vi "量程参数读取.vi"(8 "error in (no error)":errorcluster, 9 "量程下拉列表":enum16{"低量程", "高量程"}(ring), 10 "测量模式":enum16{"跨度核查", "水样测量", "零点核查", "标样核查", "加标回收"}(ring), 11 "参数下拉列表":u16(ring) items=["总磷"=1, "总氮"=2]) -> (0 "error out":errorcluster, 3 "量程切换阈值":cluster{"阈值":dbl, "标液浓度":dbl})   [LabVIEW 2016, in "斯坦道氨氮V2.lvlib"]
uses:
  <vilib>/Utility/error.llb/Error Cluster From Error Code.vi
  <vilib>/ErrorRing/Error Ring.xnode
  <vilib>/Plasmionique/MB Master/MB Master.lvlib
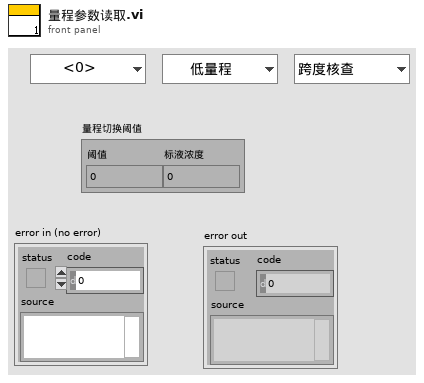
[diagram p1: front panel]
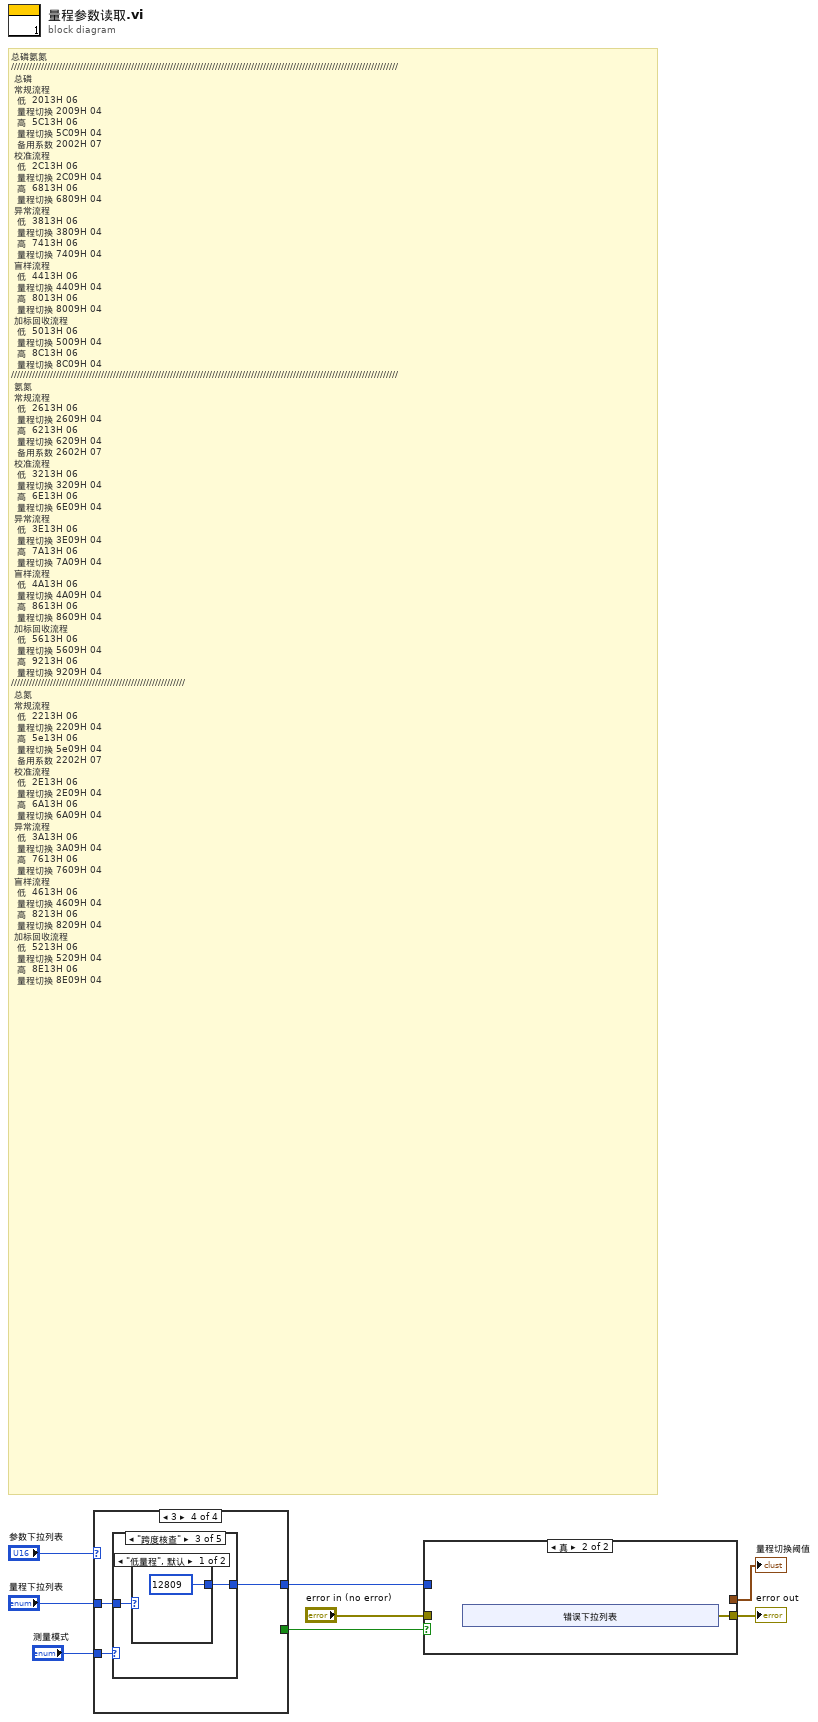
[diagram p0: block diagram]
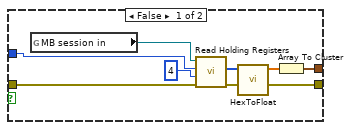
[diagram p2: hidden frame]
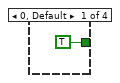
[diagram p3: hidden frame]
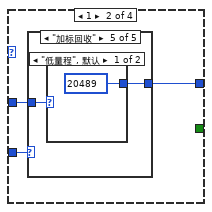
[diagram p4: hidden frame]
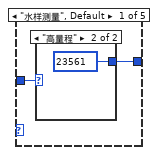
[diagram p5: hidden frame]
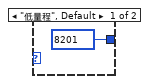
[diagram p6: hidden frame]
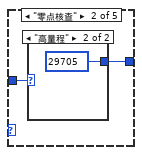
[diagram p7: hidden frame]
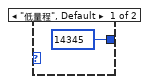
[diagram p8: hidden frame]
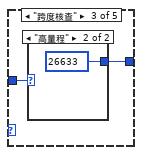
[diagram p9: hidden frame]
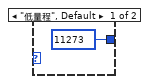
[diagram p10: hidden frame]
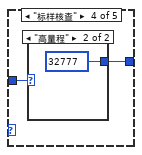
[diagram p11: hidden frame]
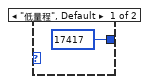
[diagram p12: hidden frame]
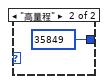
[diagram p13: hidden frame]
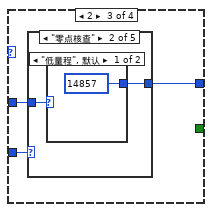
[diagram p14: hidden frame]
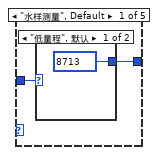
[diagram p15: hidden frame]
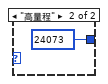
[diagram p16: hidden frame]
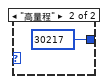
[diagram p17: hidden frame]
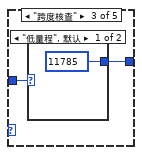
[diagram p18: hidden frame]
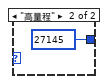
[diagram p19: hidden frame]
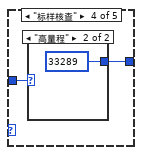
[diagram p20: hidden frame]
diagram:
  # "总磷氨氮\n/////////////////////////////////////////////////////////////////////////////////////////////////////////////////////////////////\n\t总磷\n\t常规流程\n\t\t低\t\t2013H\t06\n\t\t量程切换\t2009H\t04\n\t\t高\t\t5C13H\t06\n\t\t量程切换\t5C09H\t04\n\t\t备用系数\t2002H\t07\n\t校准流程\n\t\t低\t\t2C13H\t06\n\t\t量程切换\t2C09H\t04\n\t\t高\t\t6813H\t06\n\t\t量程切换\t6809H\t04\n\t异常流程\n\t\t低\t\t3813H\t06\n\t\t量程切换\t3809H\t04\n\t\t高\t\t7413H\t06\n\t\t量程切换\t7409H\t04\t\n\t盲样流程\n\t\t低\t\t4413H\t06\n\t\t量程切换\t4409H\t04\n\t\t高\t\t8013H\t06\n\t\t量程切换\t8009H\t04\t\n\t加标回收流程\n\t\t低\t\t5013H\t06\n\t\t量程切换\t5009H\t04\n\t\t高\t\t8C13H\t06\n\t\t量程切换\t8C09H\t04\t\n/////////////////////////////////////////////////////////////////////////////////////////////////////////////////////////////////\n\t氨氮\n\t常规流程\n\t\t低\t\t2613H\t06\n\t\t量程切换\t2609H\t04\n\t\t高\t\t6213H\t06\n\t\t量程切换\t6209H\t04\n\t\t备用系数\t2602H\t07\n\t校准流程\n\t\t低\t\t3213H\t06\n\t\t量程切换\t3209H\t04\n\t\t高\t\t6E13H\t06\n\t\t量程切换\t6E09H\t04\n\t异常流程\n\t\t低\t\t3E13H\t06\n\t\t量程切换\t3E09H\t04\n\t\t高\t\t7A13H\t06\n\t\t量程切换\t7A09H\t04\t\n\t盲样流程\n\t\t低\t\t4A13H\t06\n\t\t量程切换\t4A09H\t04\n\t\t高\t\t8613H\t06\n\t\t量程切换\t8609H\t04\t\n\t加标回收流程\n\t\t低\t\t5613H\t06\n\t\t量程切换\t5609H\t04\n\t\t高\t\t9213H\t06\n\t\t量程切换\t9209H\t04\t\n//////////////////////////////////////////////////////////\n\t总氮\n\t常规流程\n\t\t低\t\t2213H\t06\n\t\t量程切换\t2209H\t04\n\t\t高\t\t5e13H\t06\n\t\t量程切换\t5e09H\t04\n\t\t备用系数\t2202H\t07\n\t校准流程\n\t\t低\t\t2E13H\t06\n\t\t量程切换\t2E09H\t04\n\t\t高\t\t6A13H\t06\n\t\t量程切换\t6A09H\t04\n\t异常流程\n\t\t低\t\t3A13H\t06\n\t\t量程切换\t3A09H\t04\n\t\t高\t\t7613H\t06\n\t\t量程切换\t7609H\t04\t\n\t盲样流程\n\t\t低\t\t4613H\t06\n\t\t量程切换\t4609H\t04\n\t\t高\t\t8213H\t06\n\t\t量程切换\t8209H\t04\t\n\t加标回收流程\n\t\t低\t\t5213H\t06\n\t\t量程切换\t5209H\t04\n\t\t高\t\t8E13H\t06\n\t\t量程切换\t8E09H\t04"
  n1 = case shown="3" "参数下拉列表" {
    tunnel: "测量模式" -> [_ w12 w35 w58]
    tunnel: "量程下拉列表" -> [_ w11 w34 w57]
    tunnel: [_ w10 w33 w56] -> w5
    tunnel: [TRUE _ _ _] -> w2
    frame 0, Default {
    }
    frame 1 {
      n2 = case shown="\"加标回收\"" w12 {
        tunnel: w11 -> [w14 w18 w22 w26 w30]
        tunnel: [w13 w17 w21 w25 w29] -> w10
        frame "水样测量", Default {
          n3 = case shown="\"高量程\"" w14 {
            tunnel: [u16 8201 ("starting address") u16 23561 ("starting address")] -> w13
            frame "低量程", Default {
            }
            frame "高量程" {
            }
          }
        }
        frame "零点核查" {
          n4 = case shown="\"高量程\"" w18 {
            tunnel: [u16 14345 ("starting address") u16 29705 ("starting address")] -> w17
            frame "低量程", Default {
            }
            frame "高量程" {
            }
          }
        }
        frame "跨度核查" {
          n5 = case shown="\"高量程\"" w22 {
            tunnel: [u16 11273 ("starting address") u16 26633 ("starting address")] -> w21
            frame "低量程", Default {
            }
            frame "高量程" {
            }
          }
        }
        frame "标样核查" {
          n6 = case shown="\"高量程\"" w26 {
            tunnel: [u16 17417 ("starting address") u16 32777 ("starting address")] -> w25
            frame "低量程", Default {
            }
            frame "高量程" {
            }
          }
        }
        frame "加标回收" {
          n7 = case shown="\"低量程\", 默认" w30 {
            tunnel: [u16 20489 ("starting address") u16 35849 ("starting address")] -> w29
            frame "低量程", Default {
            }
            frame "高量程" {
            }
          }
        }
      }
    }
    frame 2 {
      n8 = case shown="\"零点核查\"" w35 {
        tunnel: w34 -> [w37 w41 w45 w49 w53]
        tunnel: [w36 w40 w44 w48 w52] -> w33
        frame "水样测量", Default {
          n9 = case shown="\"低量程\", 默认" w37 {
            tunnel: [u16 8713 ("starting address") u16 24073 ("starting address")] -> w36
            frame "低量程", Default {
            }
            frame "高量程" {
            }
          }
        }
        frame "零点核查" {
          n10 = case shown="\"低量程\", 默认" w41 {
            tunnel: [u16 14857 ("starting address") u16 30217 ("starting address")] -> w40
            frame "低量程", Default {
            }
            frame "高量程" {
            }
          }
        }
        frame "跨度核查" {
          n11 = case shown="\"低量程\", 默认" w45 {
            tunnel: [u16 11785 ("starting address") u16 27145 ("starting address")] -> w44
            frame "低量程", Default {
            }
            frame "高量程" {
            }
          }
        }
        frame "标样核查" {
          n12 = case shown="\"高量程\"" w49 {
            tunnel: [u16 17929 ("starting address") u16 33289 ("starting address")] -> w48
            frame "低量程", Default {
            }
            frame "高量程" {
            }
          }
        }
        frame "加标回收" {
          n13 = case shown="\"低量程\", 默认" w53 {
            tunnel: [u16 21001 ("starting address") u16 36361 ("starting address")] -> w52
            frame "低量程", Default {
            }
            frame "高量程" {
            }
          }
        }
      }
    }
    frame 3 {
      n14 = case shown="\"跨度核查\"" w58 {
        tunnel: w57 -> [w60 w64 w68 w72 w76]
        tunnel: [w59 w63 w67 w71 w75] -> w56
        frame "水样测量", Default {
          n15 = case shown="\"高量程\"" w60 {
            tunnel: [u16 9737 ("starting address") u16 25097 ("starting address")] -> w59
            frame "低量程", Default {
            }
            frame "高量程" {
            }
          }
        }
        frame "零点核查" {
          n16 = case shown="\"低量程\", 默认" w64 {
            tunnel: [u16 15881 ("starting address") u16 31241 ("starting address")] -> w63
            frame "低量程", Default {
            }
            frame "高量程" {
            }
          }
        }
        frame "跨度核查" {
          n17 = case shown="\"低量程\", 默认" w68 {
            tunnel: [u16 12809 ("starting address") u16 28169 ("starting address")] -> w67
            frame "低量程", Default {
            }
            frame "高量程" {
            }
          }
        }
        frame "标样核查" {
          n18 = case shown="\"高量程\"" w72 {
            tunnel: [u16 18963 ("starting address") u16 34323 ("starting address")] -> w71
            frame "低量程", Default {
            }
            frame "高量程" {
            }
          }
        }
        frame "加标回收" {
          n19 = case shown="\"低量程\", 默认" w76 {
            tunnel: [u16 22025 ("starting address") u16 37385 ("starting address")] -> w75
            frame "低量程", Default {
            }
            frame "高量程" {
            }
          }
        }
      }
    }
  }
  n20 = case shown="真" w2 {
    tunnel: w5 -> [w86 _]
    tunnel: "error in (no error)" -> [w84 _]
    tunnel: [w83 w87] -> w3
    tunnel: [w79 _] -> w1
    frame False {
      n21 = global read "VAR总磷总氮全局变量.vi" "MB session in"() -> (w85:refnum<class "MB_Master.lvclass">)
      n22 = call <vilib>:"Read Holding Registers.vi"("error in (no error)"=w84, "quantity"=u16 4, "starting address"=w86, "MB session in"=w85) -> ("error out"=w83:errorcluster, "Registers"=w81:u16[])  [unwired: 5 in, 1 out]
      n23 = call "HexToFloat.vi"("数组"=w81) -> ("FLOAT"=w80:sgl[])  [unwired: 10 in]
      n24 = Array To Cluster(array=w80) -> (cluster=w79:cluster{"FLOAT[0]":sgl, "FLOAT[1]":sgl})
    }
    frame True {
      n25 = xnode "错误下拉列表"() -> ("错误输出"=w87:errorcluster)
    }
  }
  "error out" <- w3
  "量程切换阈值" <- w1
